vi "parseShutterPositionFromShortStatus.vi"(8 "error in (no error)":errorcluster, 10 "shortStatus":string, 11 "DomeCommunicator in":refnum<class "DomeCommunicator.lvclass">) -> (0 "error out":errorcluster, 1 "dropoutDoorOpeningPercentage":T2, 2 "mainDoorOpeningPercentage":T1 min=0.0 max=100.0, 3 "DomeCommunicator out":refnum<class "DomeCommunicator.lvclass">, 4 "openingPercentage":T1 min=0.0 max=100.0, 5 "mainDoor":T2)   [LabVIEW 2016, in "DomeCommunicator.lvclass"]
uses:
  DomeCommunicator.lvclass
  ComTypedefs/openingStates.ctl
  IDome/domeTypedefs/openingPercentage.ctl
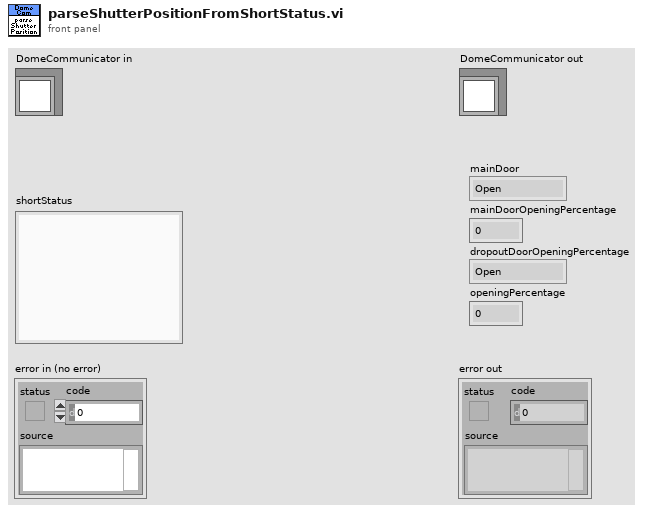
[diagram p1: front panel]
types:
  T1 = typedef "openingPercentage.ctl" = dbl
  T2 = typedef "openingStates.ctl" = enum16{"Open", "Shut", "Ajar"}
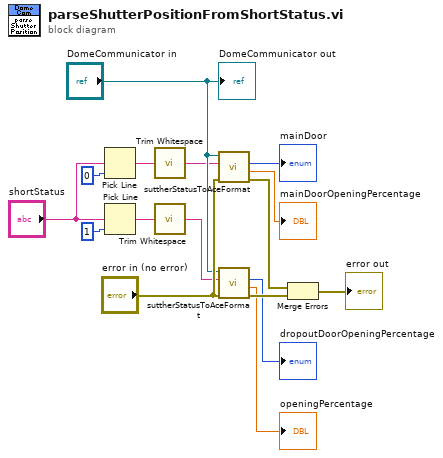
[diagram p0: block diagram]
diagram:
  n1 = Pick Line(multi-line string="shortStatus", line index=0) -> (output string=w13:string)  [unwired: 1 in]
  n2 = Pick Line(multi-line string="shortStatus", line index=1) -> (output string=w12:string)  [unwired: 1 in]
  n3 = call <vilib>:"Trim Whitespace.vi"("string"=w13) -> ("trimmed string"=w6:string)  [unwired: 1 in]
  n4 = call <vilib>:"Trim Whitespace.vi"("string"=w12) -> ("trimmed string"=w5:string)  [unwired: 1 in]
  n5 = call "suttherStatusToAceFormat.vi"("error in (no error)"="error in (no error)", "lineStatus"=w6, "DomeCommunicator in"="DomeCommunicator in") -> ("error out"=w11:errorcluster, "openingPercentage"=→"mainDoorOpeningPercentage":T1, "shutterStatus"=→"mainDoor":T2)  [unwired: 5 in, 1 out]
  n6 = call "suttherStatusToAceFormat.vi"("error in (no error)"="error in (no error)", "lineStatus"=w5, "DomeCommunicator in"="DomeCommunicator in") -> ("error out"=w10:errorcluster, "openingPercentage"=→"openingPercentage":T1, "shutterStatus"=→"dropoutDoorOpeningPercentage":T2)  [unwired: 5 in, 1 out]
  n7 = Merge Errors(w11, w10) -> (→"error out":errorcluster)
  "DomeCommunicator out" <- "DomeCommunicator in"
